vi "ROSBRIDGE TCP READ.vi"(8 "error in (no error)":errorcluster, 10 "String in":string, 11 "TCP Network Connection in":refnum<k5>) -> (0 "error out":errorcluster, 2 "String out":string, 3 "TCP Network Connection out":refnum<k5>)   [LabVIEW 2015, in "Biblioteka moduł map v3.lvlib" / "ROS.lvlib"]
uses:
  ROS.lvlib
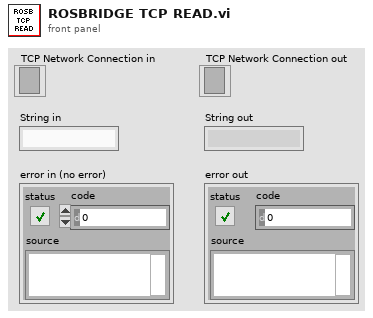
[diagram p1: front panel]
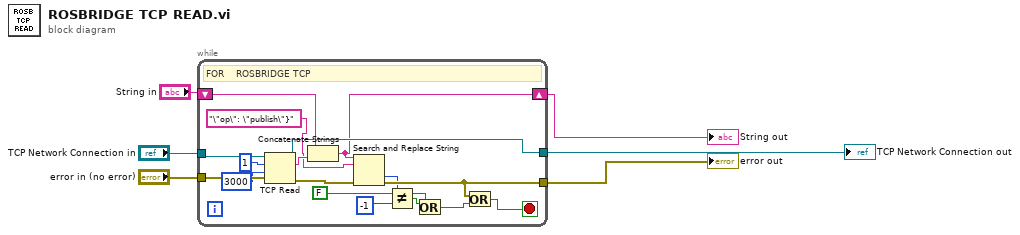
[diagram p0: block diagram]
diagram:
  n1 = while {
    shift-right: [w7] -> w2
    shift-left: "String in" -> [w17]
    tunnel: "TCP Network Connection in" -> [w23]
    tunnel: "error in (no error)" -> [w22]
    tunnel: [w15] -> w5
    tunnel: [w13] -> w6
    stop <- w14 stop-if-true
    # "FOR    ROSBRIDGE TCP"
    n2 = TCP Read(connection ID=w23, bytes to read=1, error in (no error)=w22, 9:3000 ("timeout ms (25000)")) -> (connection ID out=w15:refnum<k5>, data out=w19:string, error out=w16:errorcluster)  [unwired: 1 in]
    n3 = Concatenate Strings(w17, w19) -> (w7:string)
    n4 = Search and Replace String(input string=w7, search string="\"op\": \"publish\"}" ("op"), error in=w16) -> (offset past replacement=w10:i32, error out=w13:errorcluster)  [unwired: 5 in, 2 out]
    n5 = Not Equal?(x=w10, y=-1 ("bytes to read")) -> (x != y?=w11:bool)
    n6 = Or(x=w11, y=FALSE) -> (x .or. y?=w12:bool)
    n7 = Or(x=w13, y=w12) -> (x .or. y?=w14:bool)
  }
  "error out" <- w6
  "TCP Network Connection out" <- w5
  "String out" <- w2
